vi "GPS diagnostic.vi"() -> ()   [LabVIEW 2009]
uses:
  <vilib>/LabVIEW Targets/FPGA/cRIO/shared/nicrio_ModuleControls/nicrio_cRIO-9871_FlowControlEnum.ctl
  <vilib>/LabVIEW Targets/FPGA/cRIO/shared/nicrio_ModuleControls/nicrio_cRIO-9871_ParityEnum.ctl
  <vilib>/LabVIEW Targets/FPGA/cRIO/shared/nicrio_ModuleControls/nicrio_cRIO-9871_StopBitsEnum.ctl
  <vilib>/LabVIEW Targets/FPGA/cRIO/shared/nicrio_ModuleControls/nicrio_cRIO-9871_DataBitsEnum.ctl
  <vilib>/LabVIEW Targets/FPGA/cRIO/shared/nicrio_ModuleControls/nicrio_cRIO-9871_BaudRateEnum.ctl
  <vilib>/eio/EIOPropertyNode/EIOPropertyNode.xnode
  <vilib>/rvi/eio/nirviEIOPropertyImplementation/nirviEIOPropertyImplementation.xnode
  <vilib>/rvi/eio/common/nirviEmuTemplatePropertySet_noerrors.vi
  <vilib>/eio/EIOMethodNode/EIOMethodNode.xnode
  <vilib>/rvi/eio/nirviEIOMethodImplementation/nirviEIOMethodImplementation.xnode
  <vilib>/rvi/eio/common/nirviEmuTemplateMethod_noerrors.vi
  <vilib>/rvi/eio/common/nirviEmuClasses.ctl
  <vilib>/rvi/eio/common/nirviEmuTemplatePropertyGet_noerrors.vi
panel:
  out "SS Data 4":u8
  out "SS Timeout 4":bool
  out "SS Data 3":u8
  out "SS Timeout 3":bool
  out "SS Data 2":u8
  out "SS Timeout 2":bool
  in  "Timeout (us)":i32
  in  "Baud Rate 4":T1=enum."9600 bps" caption="Baud Rate"
  in  "Data Bits 4":T2=enum."8"
  in  "Stop Bits 4":T3
  in  "Parity 4":T4
  in  "Flow Control 4":T5
  in  "Baud Rate 3":T1=enum."9600 bps" caption="Baud Rate"
  in  "Data Bits 3":T2=enum."8"
  in  "Stop Bits 3":T3
  in  "Parity 3":T4
  in  "Flow Control 3":T5
  in  "Baud Rate 2":T1=enum."9600 bps" caption="Baud Rate"
  in  "Data Bits 2":T2=enum."8"
  in  "Stop Bits 2":T3
  in  "Parity 2":T4
  in  "Flow Control 2":T5
  out "SS Data 1":u8
  out "SS Timeout 1":bool
  in  "Baud Rate 1":T1=enum."9600 bps" caption="Baud Rate"
  in  "Data Bits 1":T2=enum."8"
  in  "Stop Bits 1":T3
  in  "Parity 1":T4
  in  "Flow Control 1":T5
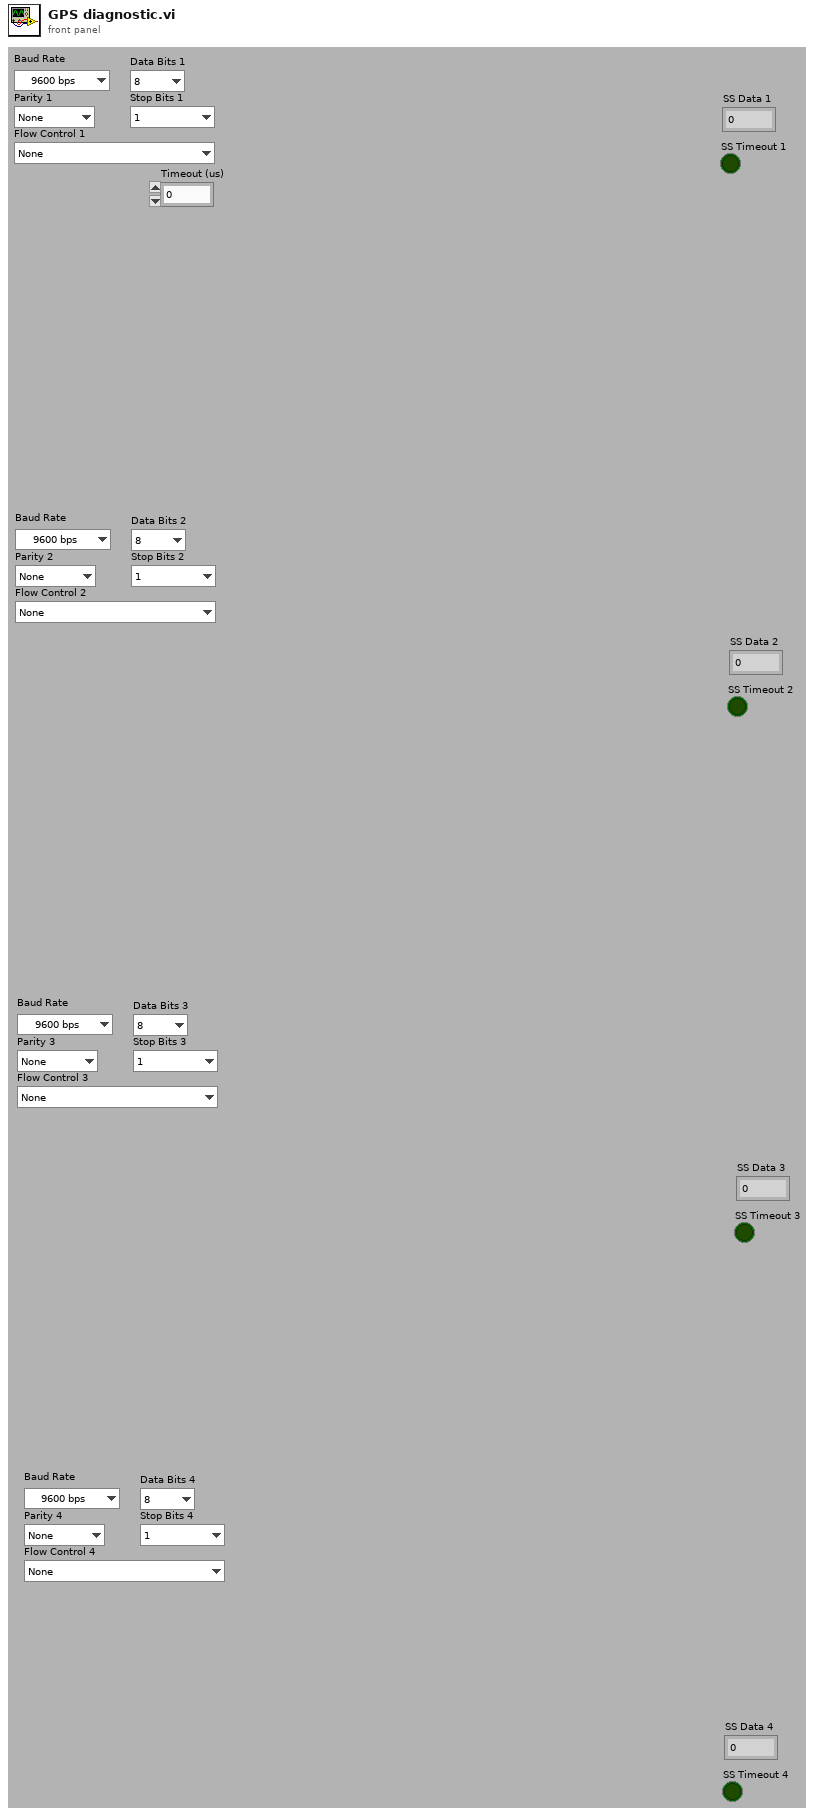
[diagram p1: front panel]
types:
  T1 = typedef "nicrio_cRIO-9871_BaudRateEnum.ctl" = enum16{"75 bps", "110 bps", "134 bps", "150 bps", "300 bps", "600 bps", "1200 bps", "1800 bps", "2400 bps", "4800 bps", "7200 bps", "9600 bps", "14.4 kbps", "19.2 kbps", "28.8 kbps", "38.4 kbps", "57.6 kbps", "115.2 kbps", "230.4 kbps", "460.8 kbps", "921.6 kbps"}
  T2 = typedef "nicrio_cRIO-9871_DataBitsEnum.ctl" = enum8{"5", "6", "7", "8"}
  T3 = typedef "nicrio_cRIO-9871_StopBitsEnum.ctl" = enum8{"1", "1.5", "2"}
  T4 = typedef "nicrio_cRIO-9871_ParityEnum.ctl" = enum8{"None", "Odd", "Even", "Mark", "Space"}
  T5 = typedef "nicrio_cRIO-9871_FlowControlEnum.ctl" = enum8{"None", "Software (XON / XOFF)", "Hardware (RTS / CTS)"}
  T6 = typedef "nirviEmuClasses.ctl" = enum16{"IO Read", "IO Write", "Method", "Property Read", "Property Write"}
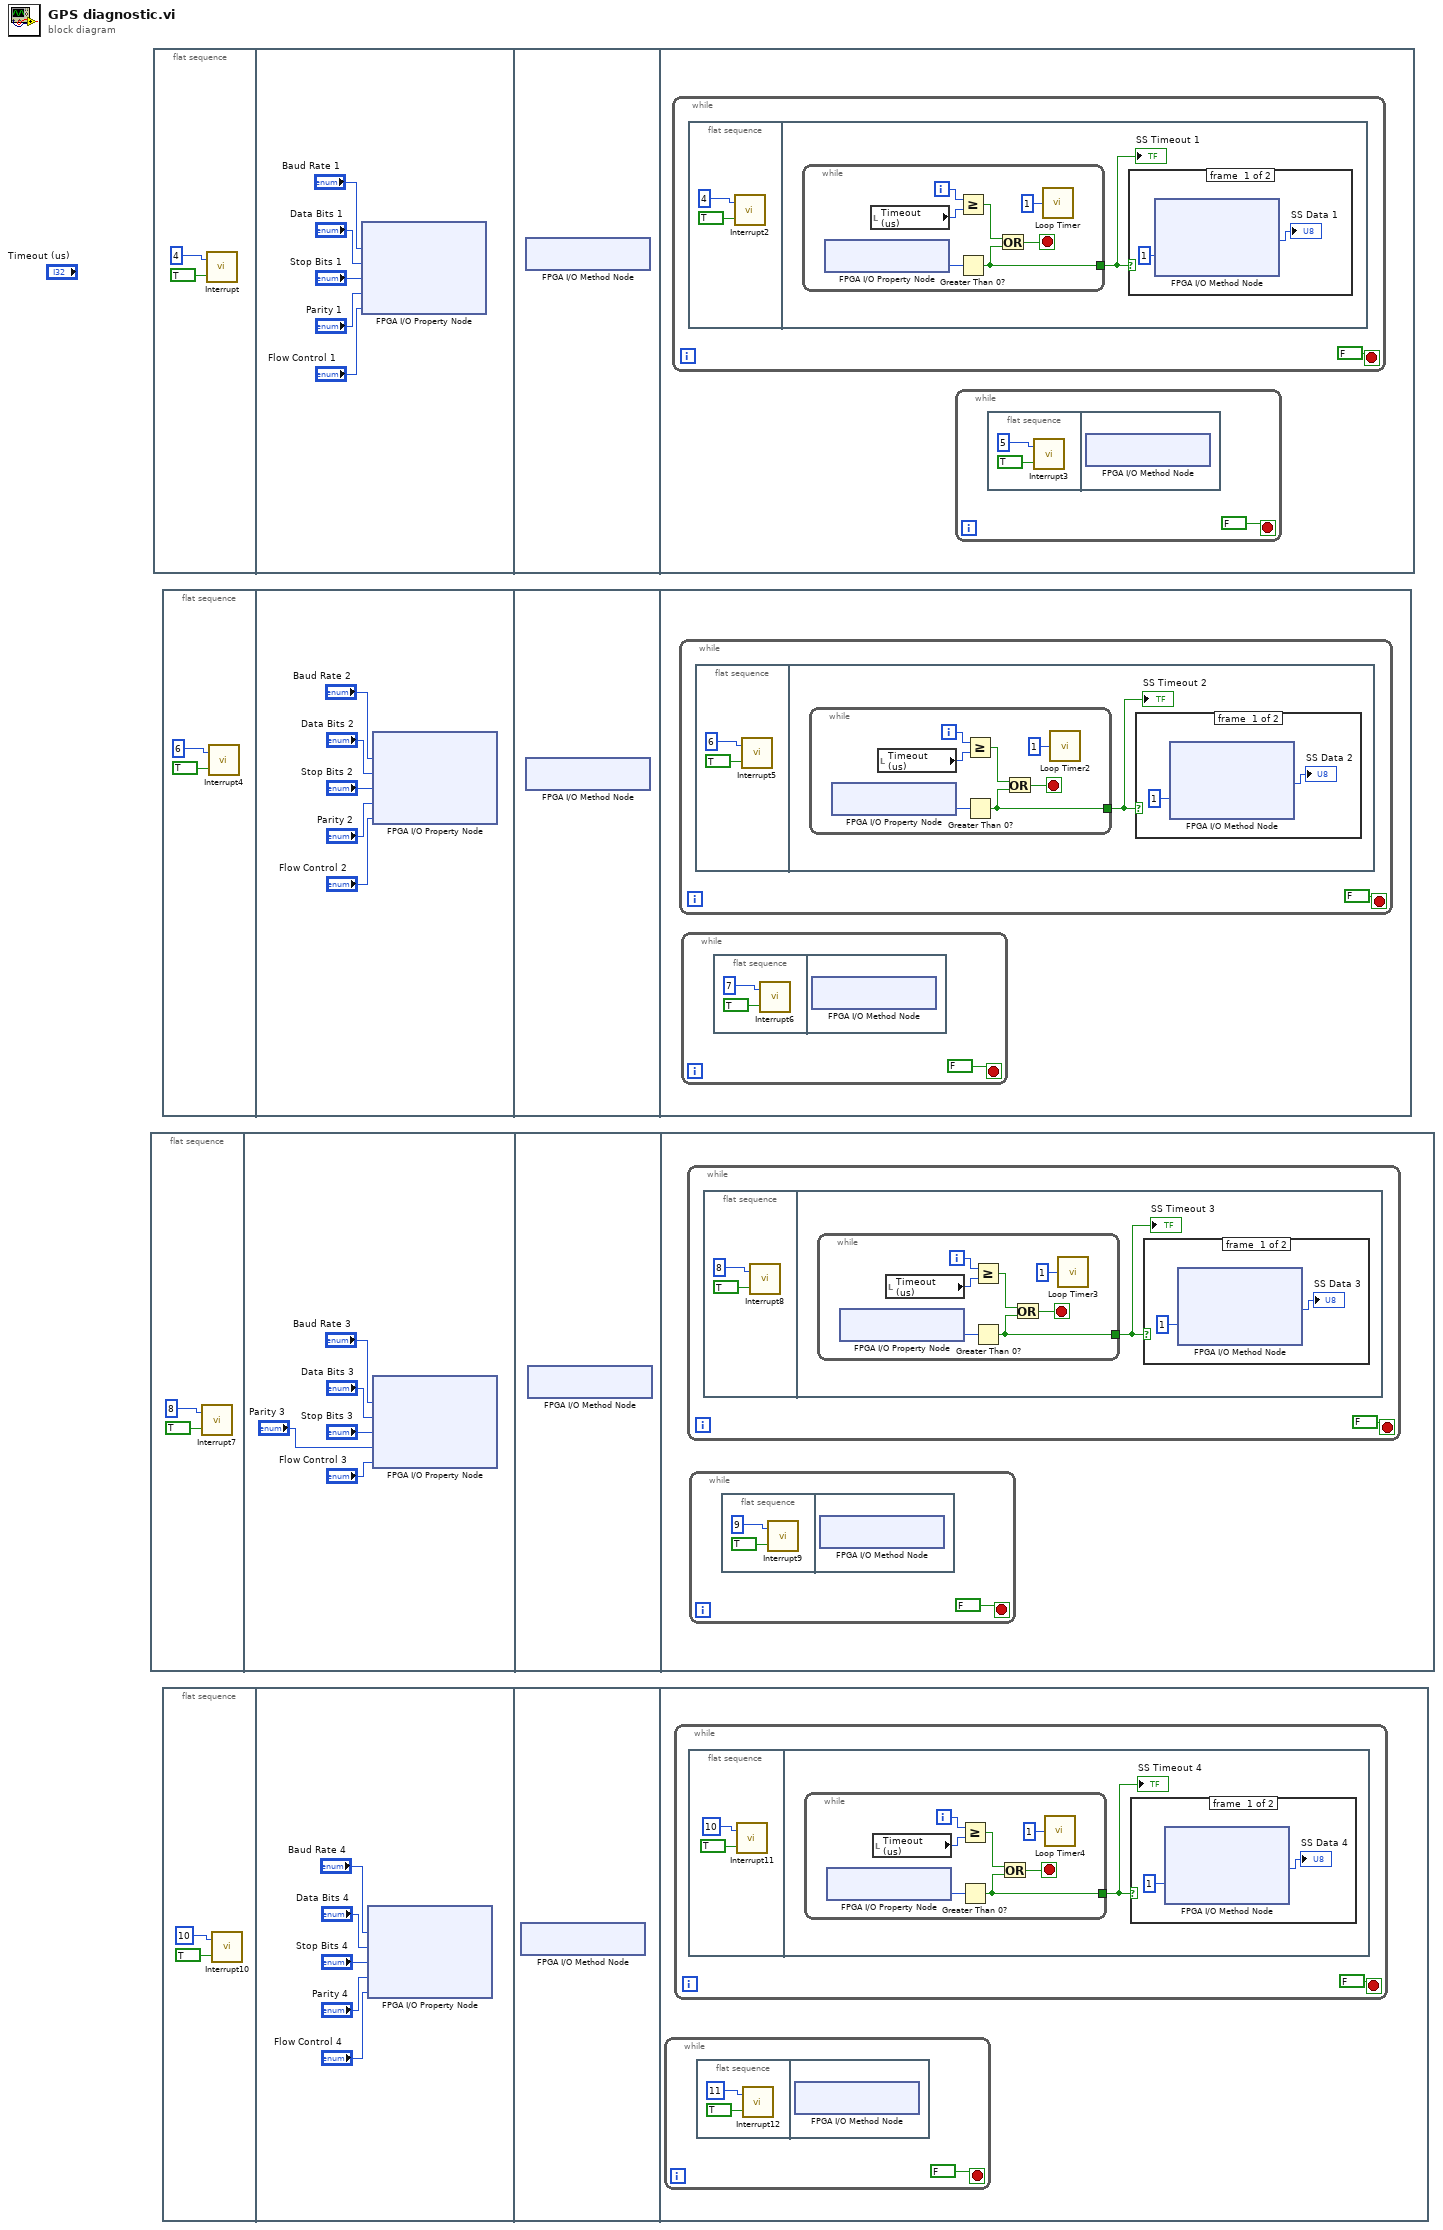
[diagram p0: block diagram]
diagram:
  n1 = flat-sequence {
    frame #0 {
      n2 = call "Interrupt7"("Wait Until Cleared"=TRUE, "IRQ Number"=u8 8 ("Port 4 wait for start IRQ")) -> ()  [unwired: 1 out]
    }
    frame #1 {
      n3 = xnode "FPGA I/O Property Node"("Baud Rate"="Baud Rate 3", "Data Bits"="Data Bits 3", "Stop Bits"="Stop Bits 3", "Parity"="Parity 3", "Flow Control"="Flow Control 3") -> ()  [unwired: 1 in, 1 out]
    }
    frame #2 {
      n4 = xnode "FPGA I/O Method Node"() -> ()  [unwired: 1 in, 1 out]
    }
    frame #3 {
      n5 = while {
        stop <- FALSE stop-if-true
        n6 = flat-sequence {
          frame #0 {
            n7 = call "Interrupt8"("Wait Until Cleared"=TRUE, "IRQ Number"=u8 8 ("Port 4 Serial Read IRQ")) -> ()  [unwired: 1 out]
          }
          frame #1 {
            n8 = while {
              tunnel: [w83] -> w47
              i -> [w88]
              stop <- w86 stop-if-true
              n9 = xnode "FPGA I/O Property Node"() -> ("Bytes at Port"=w84:u8)  [unwired: 1 in, 1 out]
              n10 = local read "Timeout (us)"() -> (w87:i32)
              n11 = Greater Or Equal?(x=w88, y=w87) -> (x >= y?=w85:bool)
              n12 = Greater Than 0?(x=w84) -> (x > 0?=w83:bool)
              n13 = Or(x=w85, y=w83) -> (x .or. y?=w86:bool)
              n14 = call "Loop Timer3"("Count(uSec)"=u32 1) -> ()  [unwired: 1 out]
            }
            "SS Timeout 3" <- w47
            n15 = case shown="False" w47 {
              frame #0 {
                n16 = xnode "FPGA I/O Method Node"("Timeout (ms)"=1) -> ("Data"=→"SS Data 3":u8)  [unwired: 1 in, 2 out]
              }
              frame #1 {
              }
            }
          }
        }
      }
      n17 = while {
        stop <- FALSE stop-if-true
        n18 = flat-sequence {
          frame #0 {
            n19 = call "Interrupt9"("Wait Until Cleared"=TRUE, "IRQ Number"=u8 9 ("Port 4 Serial Clear Rx FIFO IRQ")) -> ()  [unwired: 1 out]
          }
          frame #1 {
            n20 = xnode "FPGA I/O Method Node"() -> ()  [unwired: 1 in, 1 out]
          }
        }
      }
    }
  }
  n21 = flat-sequence {
    frame #0 {
      n22 = call "Interrupt"("Wait Until Cleared"=TRUE, "IRQ Number"=u8 4 ("Port 4 wait for start IRQ")) -> ()  [unwired: 1 out]
    }
    frame #1 {
      n23 = xnode "FPGA I/O Property Node"("Baud Rate"="Baud Rate 1", "Data Bits"="Data Bits 1", "Stop Bits"="Stop Bits 1", "Parity"="Parity 1", "Flow Control"="Flow Control 1") -> ()  [unwired: 1 in, 1 out]
    }
    frame #2 {
      n24 = xnode "FPGA I/O Method Node"() -> ()  [unwired: 1 in, 1 out]
    }
    frame #3 {
      n25 = while {
        stop <- FALSE stop-if-true
        n26 = flat-sequence {
          frame #0 {
            n27 = call "Interrupt2"("Wait Until Cleared"=TRUE, "IRQ Number"=u8 4 ("Port 4 Serial Read IRQ")) -> ()  [unwired: 1 out]
          }
          frame #1 {
            n28 = while {
              tunnel: [w205] -> w169
              i -> [w210]
              stop <- w208 stop-if-true
              n29 = xnode "FPGA I/O Property Node"() -> ("Bytes at Port"=w206:u8)  [unwired: 1 in, 1 out]
              n30 = local read "Timeout (us)"() -> (w209:i32)
              n31 = Greater Or Equal?(x=w210, y=w209) -> (x >= y?=w207:bool)
              n32 = Greater Than 0?(x=w206) -> (x > 0?=w205:bool)
              n33 = Or(x=w207, y=w205) -> (x .or. y?=w208:bool)
              n34 = call "Loop Timer"("Count(uSec)"=u32 1) -> ()  [unwired: 1 out]
            }
            "SS Timeout 1" <- w169
            n35 = case shown="False" w169 {
              frame #0 {
                n36 = xnode "FPGA I/O Method Node"("Timeout (ms)"=1) -> ("Data"=→"SS Data 1":u8)  [unwired: 1 in, 2 out]
              }
              frame #1 {
              }
            }
          }
        }
      }
      n37 = while {
        stop <- FALSE stop-if-true
        n38 = flat-sequence {
          frame #0 {
            n39 = call "Interrupt3"("Wait Until Cleared"=TRUE, "IRQ Number"=u8 5 ("Port 4 Serial Clear Rx FIFO IRQ")) -> ()  [unwired: 1 out]
          }
          frame #1 {
            n40 = xnode "FPGA I/O Method Node"() -> ()  [unwired: 1 in, 1 out]
          }
        }
      }
    }
  }
  n41 = flat-sequence {
    frame #0 {
      n42 = call "Interrupt4"("Wait Until Cleared"=TRUE, "IRQ Number"=u8 6 ("Port 4 wait for start IRQ")) -> ()  [unwired: 1 out]
    }
    frame #1 {
      n43 = xnode "FPGA I/O Property Node"("Baud Rate"="Baud Rate 2", "Data Bits"="Data Bits 2", "Stop Bits"="Stop Bits 2", "Parity"="Parity 2", "Flow Control"="Flow Control 2") -> ()  [unwired: 1 in, 1 out]
    }
    frame #2 {
      n44 = xnode "FPGA I/O Method Node"() -> ()  [unwired: 1 in, 1 out]
    }
    frame #3 {
      n45 = while {
        stop <- FALSE stop-if-true
        n46 = flat-sequence {
          frame #0 {
            n47 = call "Interrupt5"("Wait Until Cleared"=TRUE, "IRQ Number"=u8 6 ("Port 4 Serial Read IRQ")) -> ()  [unwired: 1 out]
          }
          frame #1 {
            n48 = while {
              tunnel: [w309] -> w273
              i -> [w314]
              stop <- w312 stop-if-true
              n49 = xnode "FPGA I/O Property Node"() -> ("Bytes at Port"=w310:u8)  [unwired: 1 in, 1 out]
              n50 = local read "Timeout (us)"() -> (w313:i32)
              n51 = Greater Or Equal?(x=w314, y=w313) -> (x >= y?=w311:bool)
              n52 = Greater Than 0?(x=w310) -> (x > 0?=w309:bool)
              n53 = Or(x=w311, y=w309) -> (x .or. y?=w312:bool)
              n54 = call "Loop Timer2"("Count(uSec)"=u32 1) -> ()  [unwired: 1 out]
            }
            "SS Timeout 2" <- w273
            n55 = case shown="False" w273 {
              frame #0 {
                n56 = xnode "FPGA I/O Method Node"("Timeout (ms)"=1) -> ("Data"=→"SS Data 2":u8)  [unwired: 1 in, 2 out]
              }
              frame #1 {
              }
            }
          }
        }
      }
      n57 = while {
        stop <- FALSE stop-if-true
        n58 = flat-sequence {
          frame #0 {
            n59 = call "Interrupt6"("Wait Until Cleared"=TRUE, "IRQ Number"=u8 7 ("Port 4 Serial Clear Rx FIFO IRQ")) -> ()  [unwired: 1 out]
          }
          frame #1 {
            n60 = xnode "FPGA I/O Method Node"() -> ()  [unwired: 1 in, 1 out]
          }
        }
      }
    }
  }
  n61 = flat-sequence {
    frame #0 {
      n62 = call "Interrupt10"("Wait Until Cleared"=TRUE, "IRQ Number"=u8 10 ("Port 4 wait for start IRQ")) -> ()  [unwired: 1 out]
    }
    frame #1 {
      n63 = xnode "FPGA I/O Property Node"("Baud Rate"="Baud Rate 4", "Data Bits"="Data Bits 4", "Stop Bits"="Stop Bits 4", "Parity"="Parity 4", "Flow Control"="Flow Control 4") -> ()  [unwired: 1 in, 1 out]
    }
    frame #2 {
      n64 = xnode "FPGA I/O Method Node"() -> ()  [unwired: 1 in, 1 out]
    }
    frame #3 {
      n65 = while {
        stop <- FALSE stop-if-true
        n66 = flat-sequence {
          frame #0 {
            n67 = call "Interrupt12"("Wait Until Cleared"=TRUE, "IRQ Number"=u8 11 ("Port 4 Serial Clear Rx FIFO IRQ")) -> ()  [unwired: 1 out]
          }
          frame #1 {
            n68 = xnode "FPGA I/O Method Node"() -> ()  [unwired: 1 in, 1 out]
          }
        }
      }
      n69 = while {
        stop <- FALSE stop-if-true
        n70 = flat-sequence {
          frame #0 {
            n71 = call "Interrupt11"("Wait Until Cleared"=TRUE, "IRQ Number"=u8 10 ("Port 4 Serial Read IRQ")) -> ()  [unwired: 1 out]
          }
          frame #1 {
            n72 = while {
              tunnel: [w422] -> w386
              i -> [w427]
              stop <- w425 stop-if-true
              n73 = xnode "FPGA I/O Property Node"() -> ("Bytes at Port"=w423:u8)  [unwired: 1 in, 1 out]
              n74 = local read "Timeout (us)"() -> (w426:i32)
              n75 = Greater Or Equal?(x=w427, y=w426) -> (x >= y?=w424:bool)
              n76 = Greater Than 0?(x=w423) -> (x > 0?=w422:bool)
              n77 = Or(x=w424, y=w422) -> (x .or. y?=w425:bool)
              n78 = call "Loop Timer4"("Count(uSec)"=u32 1) -> ()  [unwired: 1 out]
            }
            "SS Timeout 4" <- w386
            n79 = case shown="False" w386 {
              frame #0 {
                n80 = xnode "FPGA I/O Method Node"("Timeout (ms)"=1) -> ("Data"=→"SS Data 4":u8)  [unwired: 1 in, 2 out]
              }
              frame #1 {
              }
            }
          }
        }
      }
    }
  }
